vi "RichToFlatcif_channelcore_FIFOReference.vi"(5 "OutputClusterType":T1, 11 "InputCluster":T2) -> (3 "OutputCluster":T1)   [LabVIEW 2021, in "CIFCoreChannel_client.lvlib"]
uses:
  cif_channelcore_FIFOReference.ctl
  cif_channelcore_FIFOReference_Flat.ctl
  CIFCoreChannel_client.lvlib
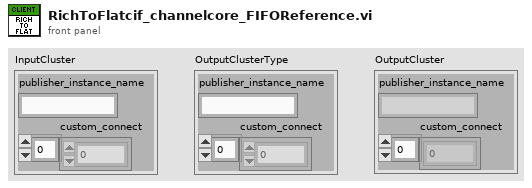
[diagram p1: front panel]
types:
  T1 = typedef "CIFCoreChannel_client.lvlib/cif_channelcore_FIFOReference_Flat.ctl" = cluster{"publisher_instance_name":string, "custom_connect":u8[]}
  T2 = typedef "CIFCoreChannel_client.lvlib/cif_channelcore_FIFOReference.ctl" = cluster{"publisher_instance_name":string, "custom_connect":u8[]}
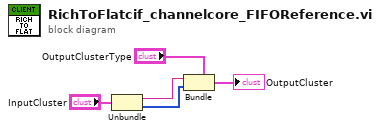
[diagram p0: block diagram]
diagram:
  n1 = Unbundle "Unbundle"("InputCluster") -> ("publisher_instance_name"=w2:string, "custom_connect"=w1:u8[])
  n2 = Bundle "Bundle"(cluster="OutputClusterType", "publisher_instance_name"=w2, "custom_connect"=w1) -> (→"OutputCluster":T1)
